vi "DeleteFiles.vi"(8 "error in (no error)":errorcluster, 11 "Path":path) -> (0 "error out":errorcluster)   [LabVIEW 2015, in "DeleteProcess.lvlib"]
uses:
  DeleteProcess.lvlib
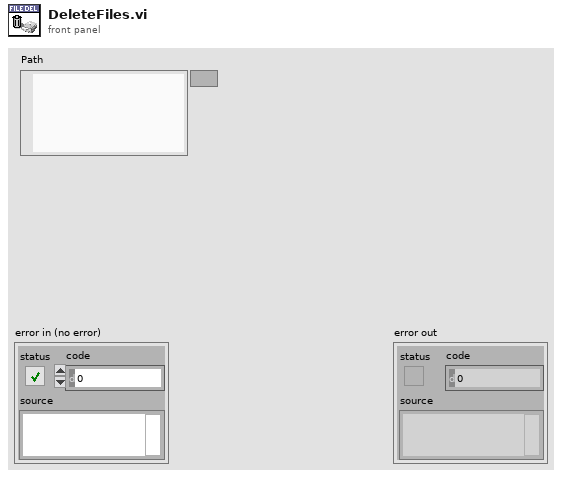
[diagram p1: front panel]
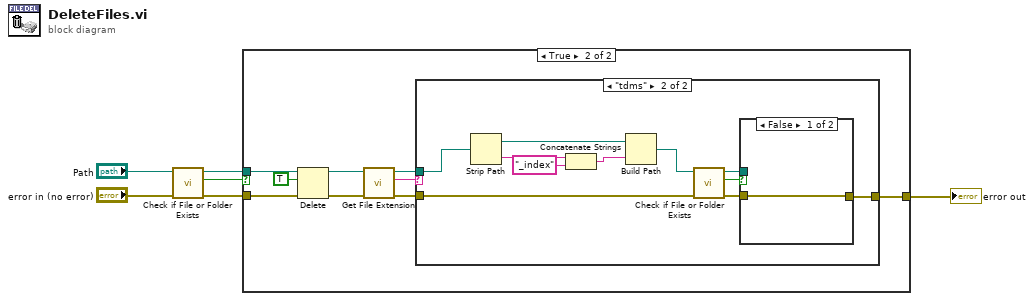
[diagram p0: block diagram]
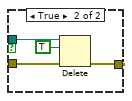
[diagram p4: hidden frame]
diagram:
  n1 = call <vilib>:"Check if File or Folder Exists.vi"("error in (no error)"="error in (no error)", "path"="Path") -> ("error out"=w4:errorcluster, "file or folder exists?"=w3:bool, "dup path"=w5:path)  [unwired: 7 in]
  n2 = case shown="True" w3 {
    tunnel: w5 -> [_ w12]
    tunnel: w4 -> [w7 w11]
    tunnel: [w7 w8] -> w2
    frame False {
    }
    frame True {
      n3 = Delete(path (use dialog)=w12, entire hierarchy (F)=TRUE, error in=w11) -> (deleted path=w10:path, error out=w9:errorcluster)  [unwired: 2 in, 1 out]
      n4 = call <vilib>:"Get File Extension.vi"("error in (no error)"=w9, "file"=w10) -> ("error out"=w14:errorcluster, "lowercase file extension"=w16:string, "dup file"=w15:path)  [unwired: 5 in, 2 out]
      n5 = case shown="\"tdms\"" w16 {
        tunnel: w15 -> [_ w28]
        tunnel: w14 -> [w17 w23]
        tunnel: [w17 w18] -> w8
        frame Default {
        }
        frame "tdms" {
          n6 = Strip Path(path=w28) -> (stripped path=w25:path, name=w27:string)
          n7 = Concatenate Strings(w27, "_index" ("string")) -> (w24:string)
          n8 = Build Path(base path=w25, name or relative path=w24) -> (appended path=w22:path)
          n9 = call <vilib>:"Check if File or Folder Exists.vi"("error in (no error)"=w23, "path"=w22) -> ("error out"=w19:errorcluster, "file or folder exists?"=w21:bool, "dup path"=w20:path)  [unwired: 7 in]
          n10 = case shown="False" w21 {
            tunnel: w20 -> [_ w32]
            tunnel: w19 -> [w29 w31]
            tunnel: [w29 w30] -> w18
            frame False {
            }
            frame True {
              n11 = Delete(path (use dialog)=w32, entire hierarchy (F)=TRUE, error in=w31) -> (error out=w30:errorcluster)  [unwired: 2 in, 2 out]
            }
          }
        }
      }
    }
  }
  "error out" <- w2
